vi "Get Control GrowInfo.vi"(8 "错误输入（无错误）":errorcluster, 11 "Ctl Ref In":refnum<vi>) -> (0 "错误输出":errorcluster, 2 "扩展信息":T1, 3 "Ctl Ref Out":refnum<vi>)   [LabVIEW 2012, in "CtrlRef.lvlib"]
uses:
  CtrlRef.lvlib
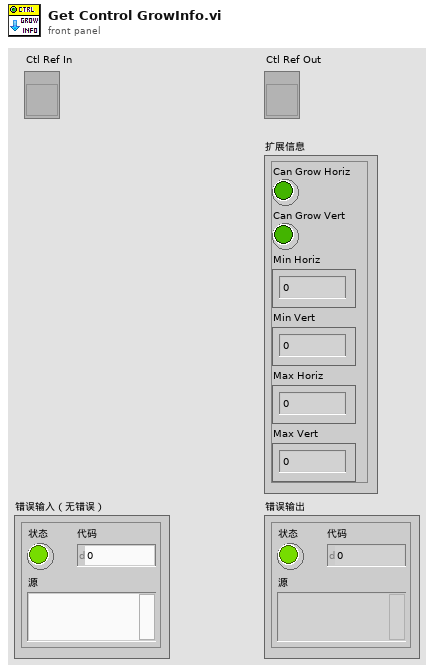
[diagram p1: front panel]
types:
  T1 = cluster{"Can Grow Horiz":bool, "Can Grow Vert":bool, "Min Horiz":i16, "Min Vert":i16, "Max Horiz":i16, "Max Vert":i16}
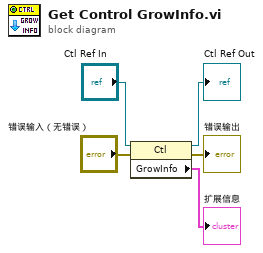
[diagram p0: block diagram]
diagram:
  n1 = property class="Ctl"(reference="Ctl Ref In", error in="错误输入（无错误）") -> (reference out=→"Ctl Ref Out":refnum<vi>, error out=→"错误输出":errorcluster, "GrowInfo"=→"扩展信息":T1)
